vi "ReadQcurve.vi"() -> (2 "Array":dbl[](array[numeric]))   [LabVIEW 2018]
uses:
  Global 2.vi
  <vilib>/Utility/file.llb/Read From Spreadsheet File (DBL).vi
panel:
  out "File name 2":string="C:\\users\\klein\\Desktop\\rssmt\\NMRave.xls"
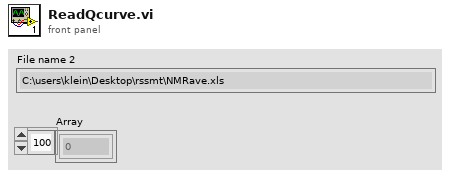
[diagram p1: front panel]
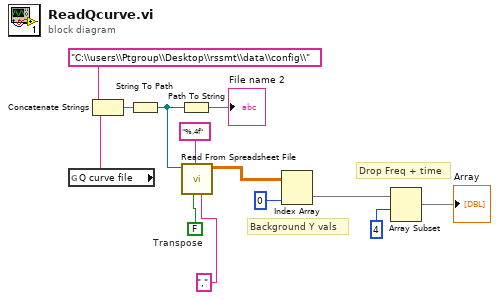
[diagram p0: block diagram]
diagram:
  w11 = FALSE  # Transpose
  # "Drop Freq + time"
  # "Background Y vals"
  n1 = global read "Global 2.vi" "Q curve file"() -> (w5:string)
  n2 = Concatenate Strings "Concatenate Strings"("C:\\users\\Ptgroup\\Desktop\\rssmt\\data\\config\\", w5) -> (w13:string)
  n3 = String To Path(string=w13) -> (path=w10:path)
  n4 = Path To String(path=w10) -> (string=→"File name 2":string)
  n5 = call-poly <vilib>:"Read From Spreadsheet File.vi"("delimiter (\\t)"=",", "transpose (no:F)"=w11, "format (%.3f)"="%.4f", "file path (dialog if empty)"=w10) -> ("all rows"=w9:dbl[][])  [unwired: 3 in, 4 out]
  n6 = Index Array(array=w9, index (col)=0) -> (element=w3:dbl[])  [unwired: 1 in]
  n7 = Array Subset(array=w3, index=4) -> (→"Array":dbl[])  [unwired: 1 in]
